vi "Read All Subordinate Object Queues.vi"(8 "error in (no error)":errorcluster, 11 "Measure Object in":refnum<class "Measure Object.lvclass">) -> (0 "error out":errorcluster, 1 "Object names":string[](array[string]), 2 "Object enqueuers":refnum<class "Message Enqueuer.lvclass">[](array[class]), 3 "Measure Object out":refnum<class "Measure Object.lvclass">)   [LabVIEW 2015, in "Measure Object.lvclass"]
uses:
  Measure Object.lvclass
  <vilib>/ActorFramework/Message Enqueuer/Message Enqueuer.lvclass
  Measure Object.lvclass/Measure Object.ctl
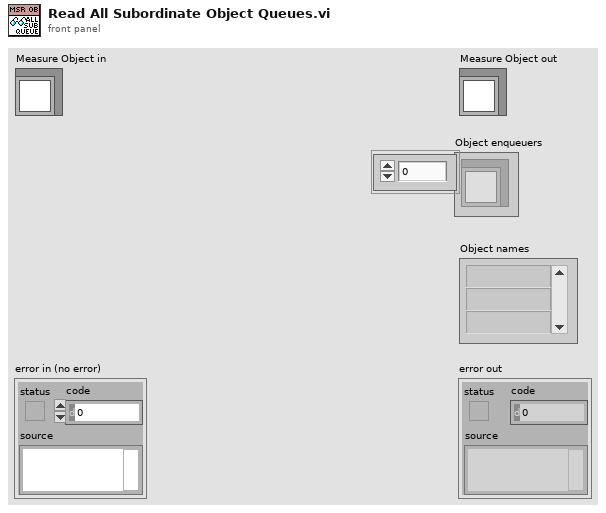
[diagram p1: front panel]
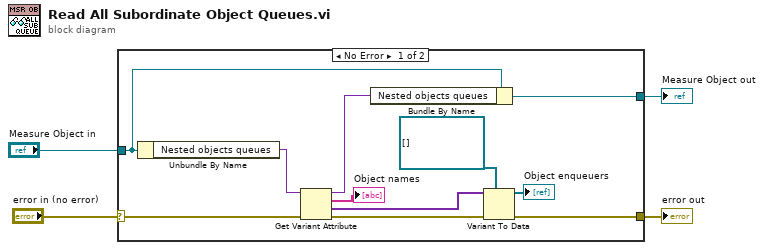
[diagram p0: block diagram]
diagram:
  n1 = case shown="No Error" "error in (no error)" {
    selector: "error in (no error)" -> [w15 w17]
    tunnel: [w7 w17] -> w3
    tunnel: [w14 w16] -> w1
    tunnel: "Measure Object in" -> [w13 w16]
    frame No Error {
      n2 = Unbundle By Name(w13) -> ("Nested objects queues"=w12:variant)
      n3 = Get Variant Attribute(Variant=w12, error in=w15) -> (duplicate Variant=w11:variant, names=→"Object names":string[], values=w10:variant[], error out=w8:errorcluster)  [unwired: 2 in]
      n4 = Bundle By Name(cluster=w13, "Nested objects queues"=w11) -> (w14:refnum<class "Measure Object.lvclass">)
      n5 = Variant To Data(error in=w8, type=refnum<class "Message Enqueuer.lvclass">[] [], Variant=w10) -> (data=→"Object enqueuers":refnum<class "Message Enqueuer.lvclass">[], error out=w7:errorcluster)
    }
    frame Error {
    }
  }
  "error out" <- w3
  "Measure Object out" <- w1
